vi "TwoFourProbe.vi"(2 "Sweeping Measurement":T9, 3 "Parameter Analizer in":T1 {"Stop Condition"."Event" items=["Value > Threshold", "Value < Threshold", "| Value | > | Threshold |", "| Value | < | Threshold |"]; "Stop Condition"."Threshold" format="%^.2e"; "Stop Condition"."Enable Delay (s)" format="%.1f"; "Sampling Time Parameters"."Sampling Time" items=["Auto (linear only)", "No Limit", "Set Limit"]; "Sampling Time Parameters"."Sampling Mode" items=["Linear", "Log10", "Log25", "Log50", "Thinned Out"]; "Sampling Time Parameters"."Hold Time (s)" format="%.4f"; "Sampling Time Parameters"."Total Sampling Time (s)" format="%.1f"; "Sampling Time Parameters"."Initial Interval (s)" format="%^.3e"; "SMU 4 - Sweeping"."Function" items=["Disabled", "Var 1", "Var 2", "Var 1'", "Constant"]; "SMU 4 - Sweeping"."Mode" items=["V", "I", "V pulse", "I  pulse", "Common"]; "SMU 4 - Sweeping"."Power \nCompliance" format="%^.2e"; "SMU 4 - Sweeping"."Compliance" format="%^.2e"; "SMU 4 - Sweeping"."Step \n(linear only)" format="%^.4e"; "SMU 4 - Sweeping"."Stop / Ratio" format="%^.4e"; "SMU 4 - Sweeping"."Start / Offset" format="%^.4e"; "SMU 3 - Sweeping"."Function" items=["Disabled", "Var 1", "Var 2", "Var 1'", "Constant"]; "SMU 3 - Sweeping"."Mode" items=["V", "I", "V pulse", "I  pulse", "Common"]; "SMU 3 - Sweeping"."Power \nCompliance" format="%^.2e"; "SMU 3 - Sweeping"."Compliance" format="%^.2e"; "SMU 3 - Sweeping"."Step \n(linear only)" format="%^.4e"; "SMU 3 - Sweeping"."Stop / Ratio" format="%^.4e"; "SMU 3 - Sweeping"."Start / Offset" format="%^.4e"; "SMU 2 - Sweeping"."Function" items=["Disabled", "Var 1", "Var 2", "Var 1'", "Constant"]; "SMU 2 - Sweeping"."Mode" items=["V", "I", "V pulse", "I  pulse", "Common"]; "SMU 2 - Sweeping"."Power \nCompliance" format="%^.2e"; "SMU 2 - Sweeping"."Compliance" format="%^.2e"; "SMU 2 - Sweeping"."Step \n(linear only)" format="%^.4e"; "SMU 2 - Sweeping"."Stop / Ratio" format="%^.4e"; "SMU 2 - Sweeping"."Start / Offset" format="%^.4e"; "SMU 1 - Sweeping"."Function" items=["Disabled", "Var 1", "Var 2", "Var 1'", "Constant"]; "SMU 1 - Sweeping"."Mode" items=["V", "I", "V pulse", "I  pulse", "Common"]; "SMU 1 - Sweeping"."Power \nCompliance" format="%^.2e"; "SMU 1 - Sweeping"."Compliance" format="%^.2e"; "SMU 1 - Sweeping"."Step \n(linear only)" format="%^.4e"; "SMU 1 - Sweeping"."Stop / Ratio" format="%^.4e"; "SMU 1 - Sweeping"."Start / Offset" format="%^.4e"; "Sweeping Time Parameters"."Long Integration Time (s)" scale=0.02..2.0; "Sweeping Time Parameters"."Short Integration Time (s)" scale=8e-05..0.00192; "Sweeping Time Parameters"."Integration Time" items=["Short", "Long"]; "Sweeping Time Parameters"."Wait Time Parameter" format="%.1f"; "SMU4 - Sampling"."Mode" items=["V", "I", "Common"]; "SMU4 - Sampling"."Compliance" format="%^.2e"; "SMU4 - Sampling"."Source" format="%^.3e"; "SMU3 - Sampling"."Mode" items=["V", "I", "Common"]; "SMU3 - Sampling"."Compliance" format="%^.2e"; "SMU3 - Sampling"."Source" format="%^.3e"; "SMU2 - Sampling"."Mode" items=["V", "I", "Common"]; "SMU2 - Sampling"."Compliance" format="%^.2e"; "SMU2 - Sampling"."Source" format="%^.3e"; "SMU1 - Sampling"."Mode" items=["V", "I", "Common"]; "SMU1 - Sampling"."Compliance" format="%^.2e"; "SMU1 - Sampling"."Source" format="%^.3e"; "Range" items=["auto", "fixed", "limited"]; "Sweep Spacing" items=["linear", "log 10", "log 25", "log 50"]}) -> (0 "Variant":variant, 1 "Parameter Analizer out":T1 {"Stop Condition"."Event" items=["Value > Threshold", "Value < Threshold", "| Value | > | Threshold |", "| Value | < | Threshold |"]; "Stop Condition"."Threshold" format="%^.2e"; "Stop Condition"."Enable Delay (s)" format="%.1f"; "Sampling Time Parameters"."Sampling Time" items=["Auto (linear only)", "No Limit", "Set Limit"]; "Sampling Time Parameters"."Sampling Mode" items=["Linear", "Log10", "Log25", "Log50", "Thinned Out"]; "Sampling Time Parameters"."Hold Time (s)" format="%.4f"; "Sampling Time Parameters"."Total Sampling Time (s)" format="%.1f"; "Sampling Time Parameters"."Initial Interval (s)" format="%^.3e"; "SMU 4 - Sweeping"."Function" items=["Disabled", "Var 1", "Var 2", "Var 1'", "Constant"]; "SMU 4 - Sweeping"."Mode" items=["V", "I", "V pulse", "I  pulse", "Common"]; "SMU 4 - Sweeping"."Power \nCompliance" format="%^.2e"; "SMU 4 - Sweeping"."Compliance" format="%^.2e"; "SMU 4 - Sweeping"."Step \n(linear only)" format="%^.4e"; "SMU 4 - Sweeping"."Stop / Ratio" format="%^.4e"; "SMU 4 - Sweeping"."Start / Offset" format="%^.4e"; "SMU 3 - Sweeping"."Function" items=["Disabled", "Var 1", "Var 2", "Var 1'", "Constant"]; "SMU 3 - Sweeping"."Mode" items=["V", "I", "V pulse", "I  pulse", "Common"]; "SMU 3 - Sweeping"."Power \nCompliance" format="%^.2e"; "SMU 3 - Sweeping"."Compliance" format="%^.2e"; "SMU 3 - Sweeping"."Step \n(linear only)" format="%^.4e"; "SMU 3 - Sweeping"."Stop / Ratio" format="%^.4e"; "SMU 3 - Sweeping"."Start / Offset" format="%^.4e"; "SMU 2 - Sweeping"."Function" items=["Disabled", "Var 1", "Var 2", "Var 1'", "Constant"]; "SMU 2 - Sweeping"."Mode" items=["V", "I", "V pulse", "I  pulse", "Common"]; "SMU 2 - Sweeping"."Power \nCompliance" format="%^.2e"; "SMU 2 - Sweeping"."Compliance" format="%^.2e"; "SMU 2 - Sweeping"."Step \n(linear only)" format="%^.4e"; "SMU 2 - Sweeping"."Stop / Ratio" format="%^.4e"; "SMU 2 - Sweeping"."Start / Offset" format="%^.4e"; "SMU 1 - Sweeping"."Function" items=["Disabled", "Var 1", "Var 2", "Var 1'", "Constant"]; "SMU 1 - Sweeping"."Mode" items=["V", "I", "V pulse", "I  pulse", "Common"]; "SMU 1 - Sweeping"."Power \nCompliance" format="%^.2e"; "SMU 1 - Sweeping"."Compliance" format="%^.2e"; "SMU 1 - Sweeping"."Step \n(linear only)" format="%^.4e"; "SMU 1 - Sweeping"."Stop / Ratio" format="%^.4e"; "SMU 1 - Sweeping"."Start / Offset" format="%^.4e"; "Sweeping Time Parameters"."Long Integration Time (s)" scale=0.02..2.0; "Sweeping Time Parameters"."Short Integration Time (s)" scale=8e-05..0.00192; "Sweeping Time Parameters"."Integration Time" items=["Short", "Long"]; "Sweeping Time Parameters"."Wait Time Parameter" format="%.1f"; "SMU4 - Sampling"."Mode" items=["V", "I", "Common"]; "SMU4 - Sampling"."Compliance" format="%^.2e"; "SMU4 - Sampling"."Source" format="%^.3e"; "SMU3 - Sampling"."Mode" items=["V", "I", "Common"]; "SMU3 - Sampling"."Compliance" format="%^.2e"; "SMU3 - Sampling"."Source" format="%^.3e"; "SMU2 - Sampling"."Mode" items=["V", "I", "Common"]; "SMU2 - Sampling"."Compliance" format="%^.2e"; "SMU2 - Sampling"."Source" format="%^.3e"; "SMU1 - Sampling"."Mode" items=["V", "I", "Common"]; "SMU1 - Sampling"."Compliance" format="%^.2e"; "SMU1 - Sampling"."Source" format="%^.3e"; "Range" items=["auto", "fixed", "limited"]; "Sweep Spacing" items=["linear", "log 10", "log 25", "log 50"]})   [LabVIEW 2014]
uses:
  Parameter Analyzer Config.ctl
  Parameter Analyzer Integration Parameters.ctl
  Parameter Analyzer SMU Sweeping.ctl
  Parameter Analyzer Sweep Spacing.ctl
  Parameter Analyzer SMU Range.ctl
  Parameter Analyzer SMU Sampling.ctl
  Parameter Analyzer Sampling Parameters.ctl
  Parameter Analyzer Stop Sampling Conditions.ctl
panel:
  # "LICENSED MATERIALS – PROPERTY OF IBM\nCopyright IBM Corp. 2016,\nALL RIGHTS RESERVED"
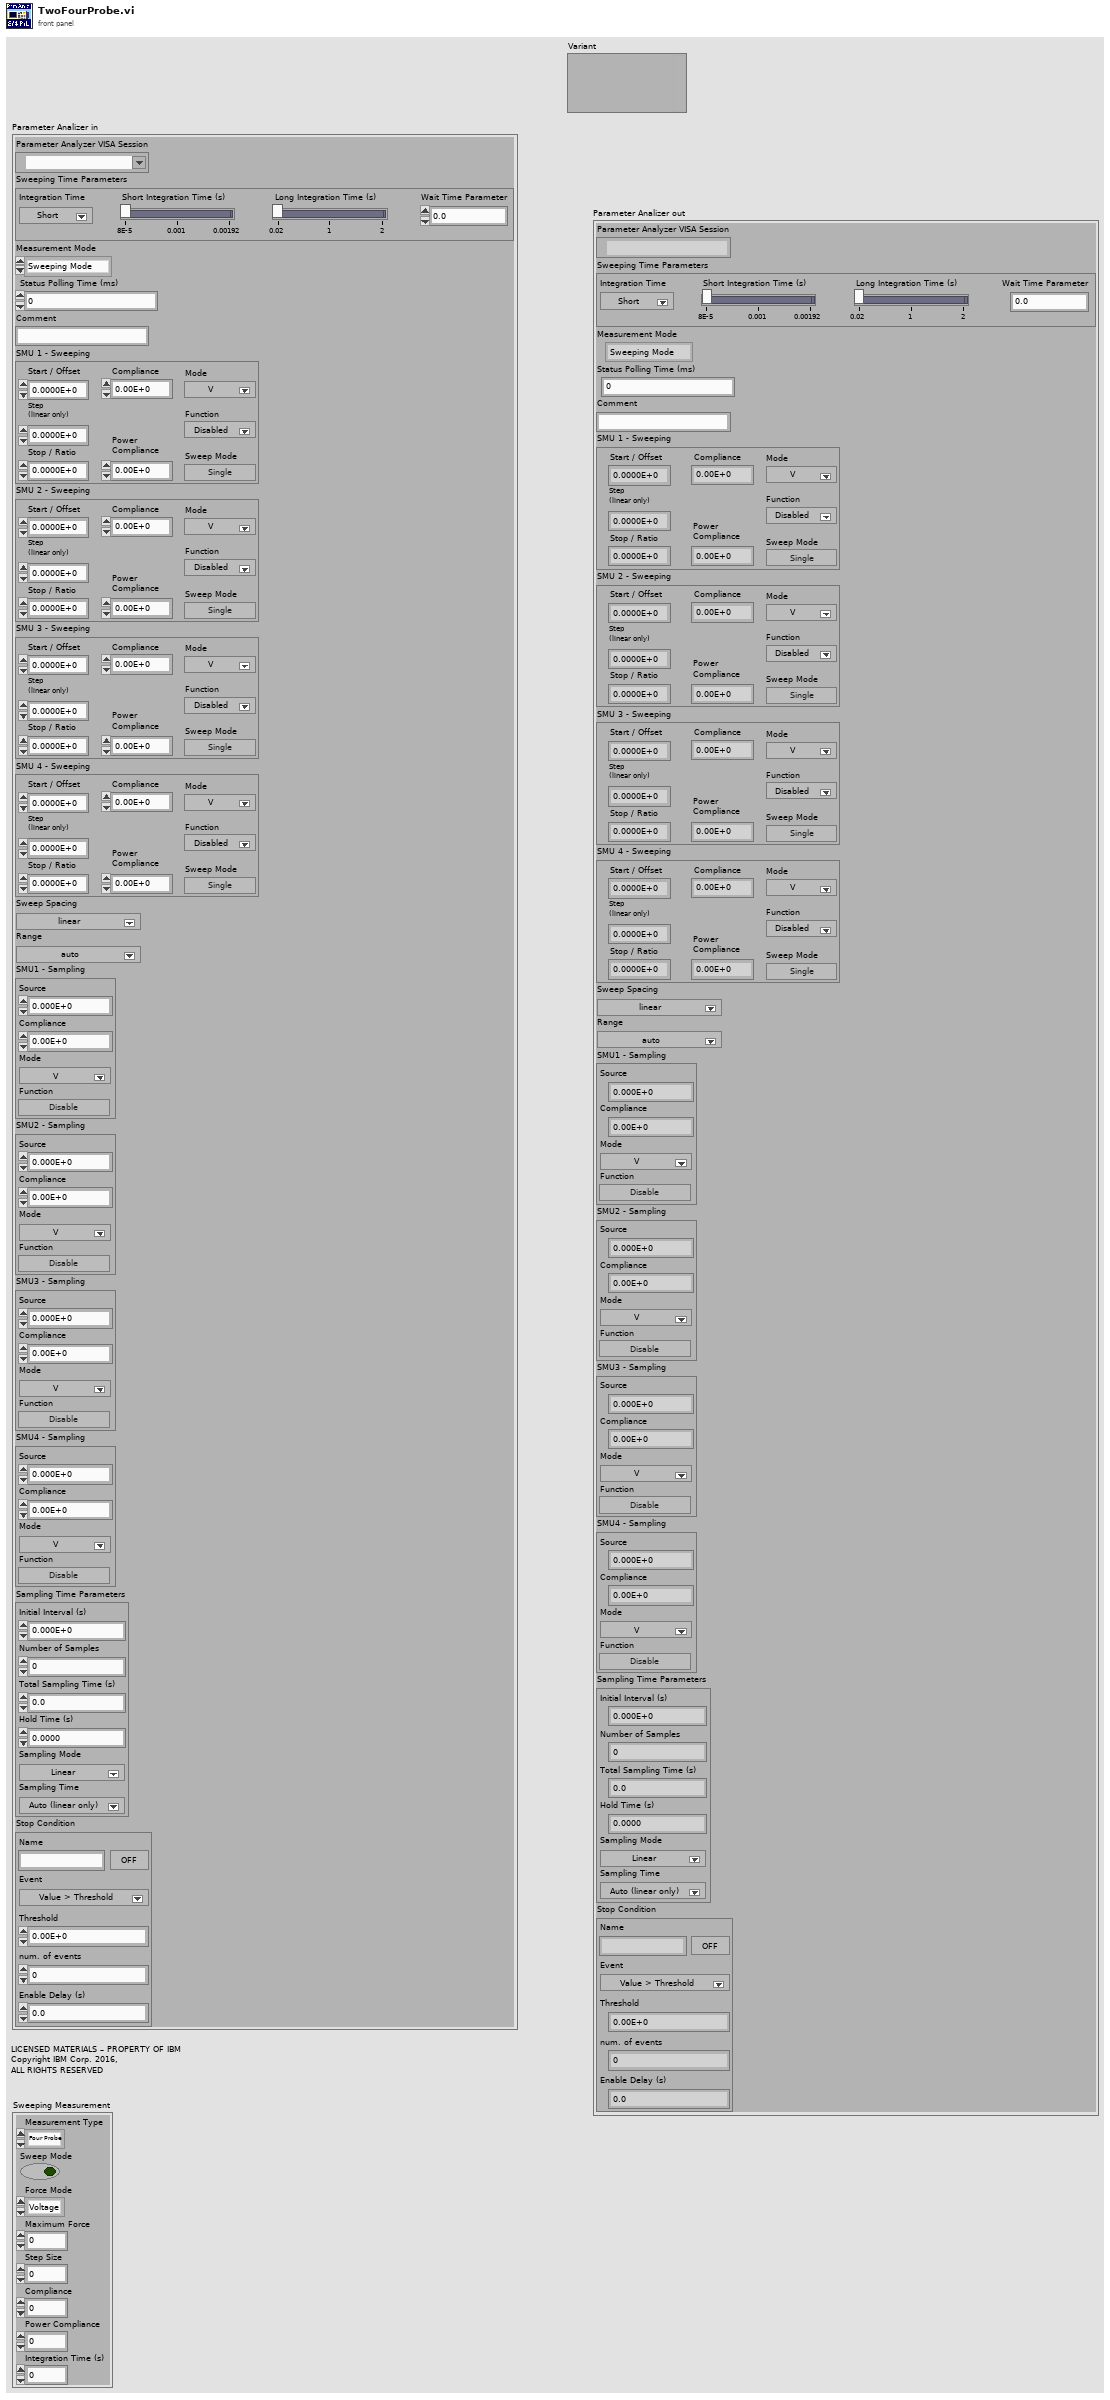
[diagram p1: front panel]
types:
  T1 = typedef "Parameter Analyzer Config.ctl" = cluster{"Parameter Analyzer VISA Session":refnum<visa-resource-name>, "Sweeping Time Parameters":T2, "Acquisition Mode":enum32{"Sweeping Mode", "Sampling Mode"}, "Status Polling Time (ms)":u32, "Comment":string, "SMU 1 - Sweeping":T3, "SMU 2 - Sweeping":T3, "SMU 3 - Sweeping":T3, "SMU 4 - Sweeping":T3, "Sweep Spacing":T4, "Range":T5, "SMU1 - Sampling":T6, "SMU2 - Sampling":T6, "SMU3 - Sampling":T6, "SMU4 - Sampling":T6, "Sampling Time Parameters":T7, "Stop Condition":T8}
  T2 = typedef "Parameter Analyzer Integration Parameters.ctl" = cluster{"Integration Time":u32, "Short Integration Time (s)":dbl, "Long Integration Time (s)":dbl, "Wait Time Parameter":dbl}
  T3 = typedef "Parameter Analyzer SMU Sweeping.ctl" = cluster{"Start / Offset":dbl, "Stop / Ratio":dbl, "Step \n(linear only)":dbl, "Compliance":dbl, "Power \nCompliance":dbl, "Mode":u32, "Function":i32, "Sweep Mode":bool}
  T4 = typedef "Parameter Analyzer Sweep Spacing.ctl" = u16
  T5 = typedef "Parameter Analyzer SMU Range.ctl" = u16
  T6 = typedef "Parameter Analyzer SMU Sampling.ctl" = cluster{"Source":dbl, "Compliance":dbl, "Mode":u32, "Function":bool}
  T7 = typedef "Parameter Analyzer Sampling Parameters.ctl" = cluster{"Initial Interval (s)":dbl, "Number of Samples":i32, "Total Sampling Time (s)":dbl, "Hold Time (s)":dbl, "Sampling Mode":i32, "Sampling Time":i32}
  T8 = typedef "Parameter Analyzer Stop Sampling Conditions.ctl" = cluster{"Enable Delay (s)":dbl, "Name":string, "Threshold":dbl, "num. of events":i32, "Event":i32, "Stop Condition Enable":bool}
  T9 = cluster{"Measurement Type":enum32{"Four Probe", "Two Probe"}, "Sweep Mode":bool, "Force Mode":enum32{"Voltage", "Current"}, "Maximum Force":dbl, "Step Size":dbl, "Compliance":dbl, "Power Compliance":dbl, "Integration Time (s)":dbl}
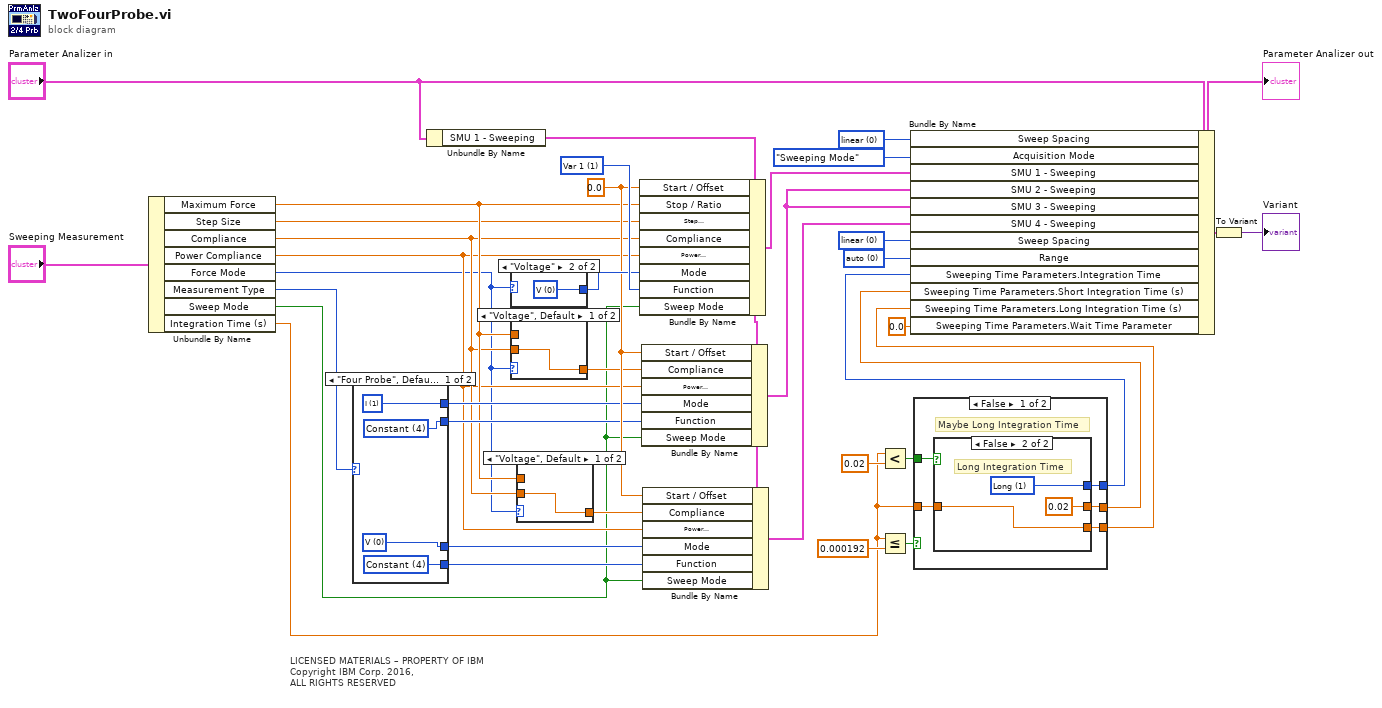
[diagram p0: block diagram]
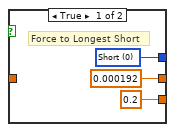
[diagram p2: hidden frame]
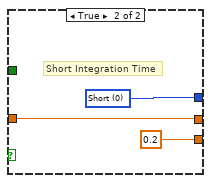
[diagram p3: hidden frame]
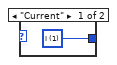
[diagram p4: hidden frame]
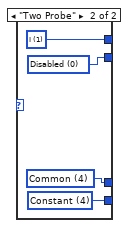
[diagram p5: hidden frame]
diagram:
  w35 = 1 items=["Disabled", "Var 1", "Var 2", "Var 1'", "Constant"] ("Function")
  w26 = u16 0 items=["linear", "log 10", "log 25", "log 50"] ("Sweep Spacing")
  w25 = u16 0 items=["auto", "fixed", "limited"] ("Range")
  w10 = u16 0 items=["linear", "log 10", "log 25", "log 50"] ("Sweep Spacing")
  w22 = 0.0 ("Start / Offset")
  # "LICENSED MATERIALS – PROPERTY OF IBM\nCopyright IBM Corp. 2016,\nALL RIGHTS RESERVED"
  n1 = Unbundle By Name("Sweeping Measurement") -> ("Maximum Force"=w8:dbl, "Step Size"=w7:dbl, "Compliance"=w6:dbl, "Power Compliance"=w5:dbl, "Force Mode"=w3:enum32{"Voltage", "Current"}, "Measurement Type"=w1:enum32{"Four Probe", "Two Probe"}, "Sweep Mode"=w2:bool, "Integration Time (s)"=w4:dbl)
  n2 = case shown="\"Four Probe\", Default" w1 {
    tunnel: [w39 w43] -> w14
    tunnel: [w38 w42] -> w13
    tunnel: [w41 w45] -> w12
    tunnel: [w40 w44] -> w11
    frame "Four Probe", Default {
      w38 = 4 items=["Disabled", "Var 1", "Var 2", "Var 1'", "Constant"] ("Function")
      w39 = 4 items=["Disabled", "Var 1", "Var 2", "Var 1'", "Constant"] ("Function")
      w40 = u32 0 items=["V", "I", "V pulse", "I  pulse", "Common"] ("Mode")
      w41 = u32 1 items=["V", "I", "V pulse", "I  pulse", "Common"] ("Mode")
    }
    frame "Two Probe" {
      w42 = 4 items=["Disabled", "Var 1", "Var 2", "Var 1'", "Constant"] ("Function")
      w43 = 0 items=["Disabled", "Var 1", "Var 2", "Var 1'", "Constant"] ("Function")
      w44 = u32 4 items=["V", "I", "V pulse", "I  pulse", "Common"] ("Mode")
      w45 = u32 1 items=["V", "I", "V pulse", "I  pulse", "Common"] ("Mode")
    }
  }
  n3 = Unbundle By Name("Parameter Analizer in") -> ("SMU 1 - Sweeping"=w16:T3)
  n4 = case shown="\"Voltage\"" w3 {
    tunnel: [w46 w47] -> w23
    frame "Current" {
      w46 = u32 1 items=["V", "I", "V pulse", "I  pulse", "Common"] ("Mode")
    }
    frame "Voltage" {
      w47 = u32 0 items=["V", "I", "V pulse", "I  pulse", "Common"] ("Mode")
    }
  }
  n5 = case shown="\"Voltage\", Default" w3 {
    tunnel: w8 -> [_ w49]
    tunnel: [w48 w49] -> w20
    tunnel: w6 -> [w48 _]
    frame "Voltage", Default {
    }
    frame "Current" {
    }
  }
  n6 = case shown="\"Voltage\", Default" w3 {
    tunnel: w8 -> [_ w51]
    tunnel: [w50 w51] -> w21
    tunnel: w6 -> [w50 _]
    frame "Voltage", Default {
    }
    frame "Current" {
    }
  }
  n7 = Bundle By Name(cluster=w16, "Start / Offset"=w22, "Stop / Ratio"=w8, "Step \n(linear only)"=w7, "Compliance"=w6, "Power \nCompliance"=w5, "Mode"=w23, "Function"=w35, "Sweep Mode"=w2) -> (w17:T3)
  n8 = Bundle By Name(cluster=w16, "Start / Offset"=w22, "Compliance"=w20, "Power \nCompliance"=w5, "Mode"=w12, "Function"=w14, "Sweep Mode"=w2) -> (w19:T3)
  n9 = Bundle By Name(cluster=w16, "Start / Offset"=w22, "Compliance"=w21, "Power \nCompliance"=w5, "Mode"=w11, "Function"=w13, "Sweep Mode"=w2) -> (w18:T3)
  n10 = Less?(x=w4, y=0.02) -> (x < y?=w34:bool)
  n11 = Less Or Equal?(x=w4, y=0.000192) -> (x <= y?=w33:bool)
  n12 = case shown="False" w33 {
    tunnel: w34 -> [w56 _]
    tunnel: [w55 w65] -> w30
    tunnel: w4 -> [w54 w64]
    tunnel: [w53 w64] -> w31
    tunnel: [w52 0.2 ("Wait Time Parameter")] -> w32
    frame False {
      # "Maybe Long Integration Time"
      n13 = case shown="False" w56 {
        tunnel: [w59 w60] -> w55
        tunnel: w54 -> [_ w61]
        tunnel: [0.000192 ("Wait Time Parameter") 0.02 ("Wait Time Parameter")] -> w53
        tunnel: [0.2 ("Wait Time Parameter") w61] -> w52
        frame True {
          w59 = u32 0 items=["Short", "Long"] ("Integration Time")
          # "Force to Longest Short"
        }
        frame False {
          w60 = u32 1 items=["Short", "Long"] ("Integration Time")
          # "Long Integration Time"
        }
      }
    }
    frame True {
      w65 = u32 0 items=["Short", "Long"] ("Integration Time")
      # "Short Integration Time"
    }
  }
  n14 = Bundle By Name(cluster="Parameter Analizer in", "Sweep Spacing"=w10, "Acquisition Mode"=enum32{"Sweeping Mode", "Sampling Mode"}."Sweeping Mode" ("Configuration.Acquisition Mode"), "SMU 1 - Sweeping"=w17, "SMU 2 - Sweeping"=w19, "SMU 3 - Sweeping"=w19, "SMU 4 - Sweeping"=w18, "Sweep Spacing"=w26, "Range"=w25, "Sweeping Time Parameters.Integration Time"=w30, "Sweeping Time Parameters.Short Integration Time (s)"=w31, "Sweeping Time Parameters.Long Integration Time (s)"=w32, "Sweeping Time Parameters.Wait Time Parameter"=0.0 ("Long Integration Time (s)")) -> (w37:T1)
  "Parameter Analizer out" <- w37
  n15 = To Variant(anything=w37) -> (Variant=→"Variant":variant)
